vi "New File.vi"(8 "error in":errorcluster, 11 "File Observer in":refnum<class "File Observer.lvclass">) -> (0 "error out":errorcluster, 2 "Exceeded":bool, 3 "File Observer out":refnum<class "File Observer.lvclass">)   [LabVIEW 2014, in "File Observer.lvclass"]
doc: "Housekeeping to see if the current file has exceeded the maximum file size indicated by the caller. If it has, the variable Exceeded == TRUE."
uses:
  File Observer.lvclass
  File Observer.lvclass/File Observer.ctl
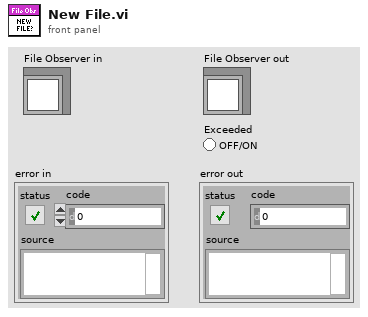
[diagram p1: front panel]
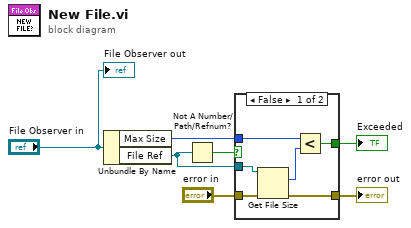
[diagram p0: block diagram]
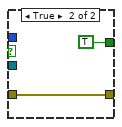
[diagram p2: hidden frame]
diagram:
  n1 = Unbundle By Name("File Observer in") -> ("Max Size"=w3:i64, "File Ref"=w5:refnum<file>)
  n2 = Not A Number/Path/Refnum?(number/path/refnum=w5) -> (NaN/Path/Refnum?=w1:bool)
  n3 = case shown="False" w1 {
    tunnel: [w13 w15] -> w7
    tunnel: "error in" -> [w12 w15]
    tunnel: w5 -> [w11 _]
    tunnel: [w10 TRUE] -> w4
    tunnel: w3 -> [w9 _]
    frame False {
      n4 = Get File Size(file=w11, error in=w12) -> (size (in bytes)=w8:i64, 0:w13:errorcluster)  [unwired: 1 out]
      n5 = Less?(x=w9, y=w8) -> (x < y?=w10:bool)
    }
    frame True {
    }
  }
  "error out" <- w7
  "Exceeded" <- w4
  "File Observer out" <- "File Observer in"
